vi "string2vec.vi"(10 "Default (nan,nan,nan)":cluster{"X":dbl, "Y":dbl, "Z":dbl}, 11 "input string":string) -> (0 "isDefault":cluster{bool, bool, bool}, 3 "output":cluster{"X":dbl, "Y":dbl, "Z":dbl})   [LabVIEW 2015]
uses:
  flipYZdbl.vi
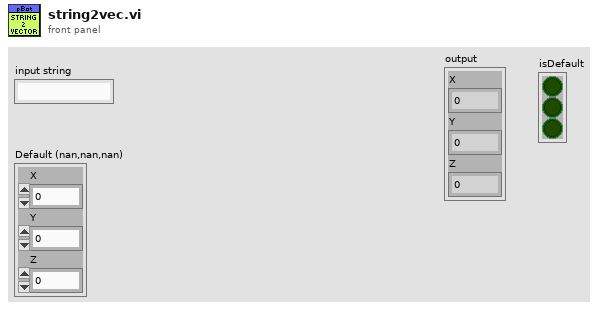
[diagram p1: front panel]
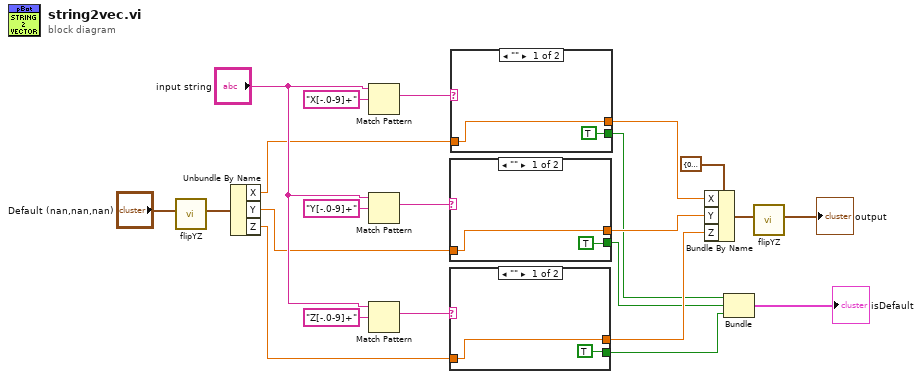
[diagram p0: block diagram]
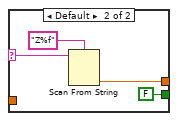
[diagram p2: hidden frame]
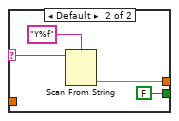
[diagram p3: hidden frame]
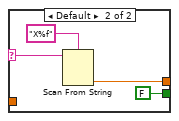
[diagram p4: hidden frame]
diagram:
  n1 = call-poly "flipYZ.vi"("pointIn"="Default (nan,nan,nan)") -> ("pointOut"=w14:cluster{"X":dbl, "Y":dbl, "Z":dbl})  [unwired: 10 in]
  n2 = Unbundle By Name(w14) -> ("X"=w6:dbl, "Y"=w13:dbl, "Z"=w12:dbl)
  n3 = Match Pattern(string="input string", regular expression="X[-.0-9]+") -> (match substring=w19:string)  [unwired: 1 in, 3 out]
  n4 = Match Pattern(string="input string", regular expression="Y[-.0-9]+") -> (match substring=w18:string)  [unwired: 1 in, 3 out]
  n5 = Match Pattern(string="input string", regular expression="Z[-.0-9]+") -> (match substring=w17:string)  [unwired: 1 in, 3 out]
  n6 = case shown="\"\"" w18 {
    selector: w18 -> [_ w27]
    tunnel: w13 -> [w24 _]
    tunnel: [w24 w26] -> w9
    tunnel: [TRUE FALSE] -> w4
    frame "" {
    }
    frame Default {
      n7 = Scan From String(format string="Y%f", input string=w27) -> (output 1=w26:dbl)  [unwired: 3 in, 3 out]
    }
  }
  n8 = case shown="\"\"" w17 {
    selector: w17 -> [_ w33]
    tunnel: w12 -> [w30 _]
    tunnel: [w30 w32] -> w8
    tunnel: [TRUE FALSE] -> w3
    frame "" {
    }
    frame Default {
      n9 = Scan From String(format string="Z%f", input string=w33) -> (output 1=w32:dbl)  [unwired: 3 in, 3 out]
    }
  }
  n10 = case shown="\"\"" w19 {
    selector: w19 -> [_ w39]
    tunnel: w6 -> [w36 _]
    tunnel: [w36 w38] -> w10
    tunnel: [TRUE FALSE] -> w2
    frame "" {
    }
    frame Default {
      n11 = Scan From String(format string="X%f", input string=w39) -> (output 1=w38:dbl)  [unwired: 3 in, 3 out]
    }
  }
  n12 = Bundle By Name(cluster=cluster{"X":dbl, "Y":dbl, "Z":dbl} {"X"=0.0, "Y"=0.0, "Z"=0.0} ("Offset (0,0,0) 2"), "X"=w10, "Y"=w9, "Z"=w8) -> (w7:cluster{"X":dbl, "Y":dbl, "Z":dbl})
  n13 = Bundle(w2, w4, w3) -> (→"isDefault":cluster{bool, bool, bool})  [unwired: 1 in]
  n14 = call-poly "flipYZ.vi"("pointIn"=w7) -> ("pointOut"=→"output":cluster{"X":dbl, "Y":dbl, "Z":dbl})  [unwired: 10 in]
